vi "DatatoString.vi"(4 "Decimal Places (SI)":i32=6, 6 "Unit Modifier":enum16{"None", "RMS", "P-to-P"}(ring), 7 "SI Notation":bool, 9 "Units":string, 10 "Decimal Places (non-SI)":i32, 11 "Number":dbl format="%.6p") -> (3 "String":string)   [LabVIEW 2011]
panel:
  out "String 2":string
  # "P-to-P: Peak-to-Peak"
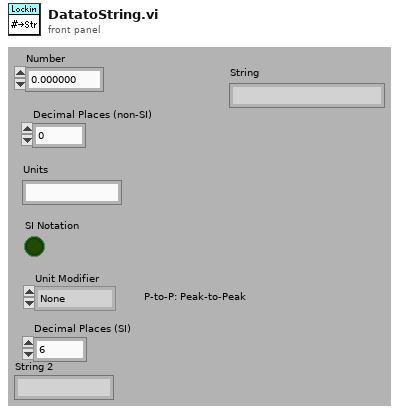
[diagram p1: front panel]
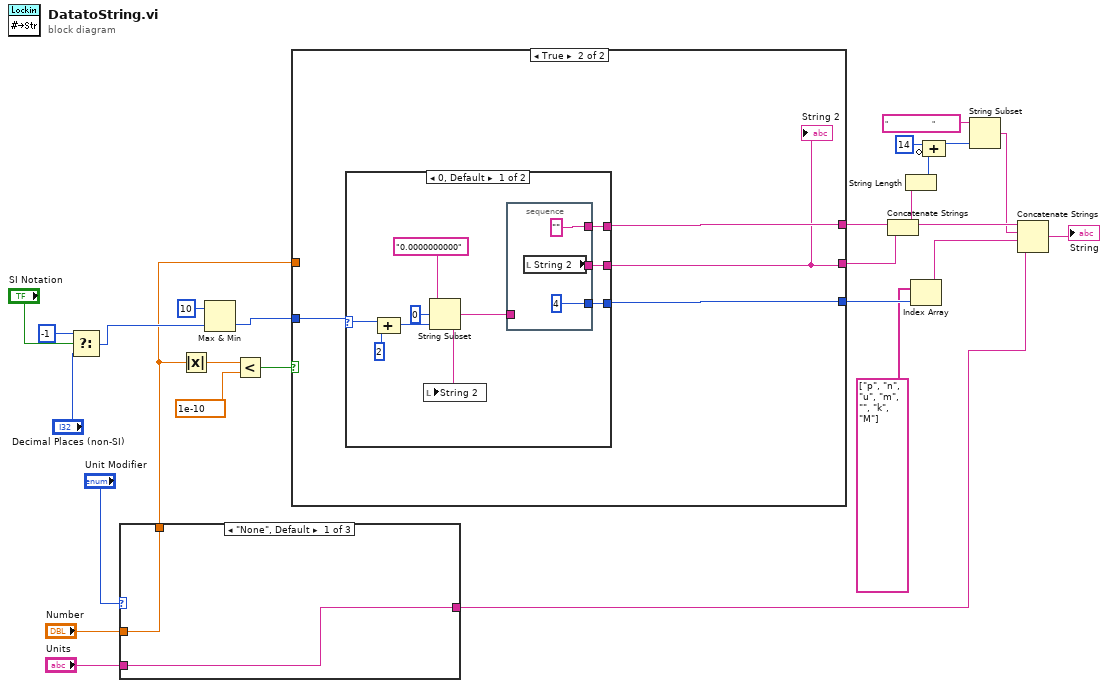
[diagram p0: block diagram]
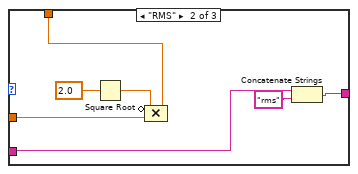
[diagram p2: hidden frame]
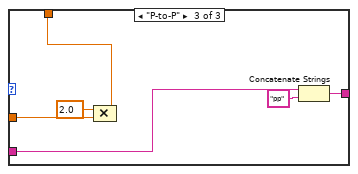
[diagram p3: hidden frame]
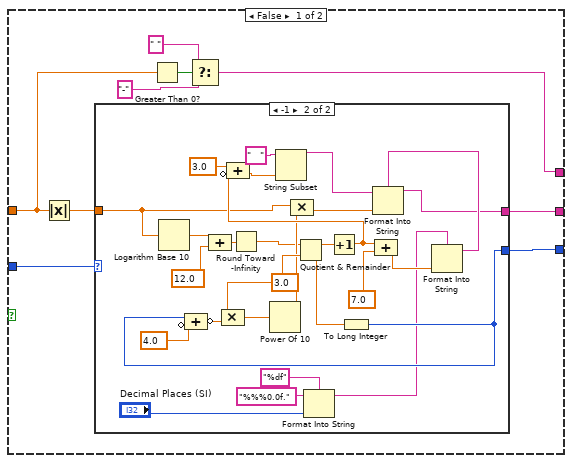
[diagram p4: hidden frame]
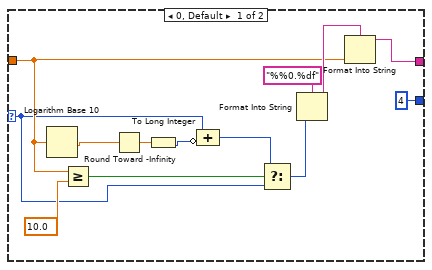
[diagram p5: hidden frame]
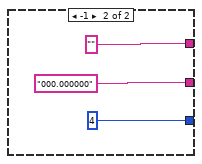
[diagram p6: hidden frame]
diagram:
  n1 = Select(t=-1, s="SI Notation", f="Decimal Places (non-SI)") -> (s? t:f=w7:i32)
  n2 = case shown="\"None\", Default" "Unit Modifier" {
    tunnel: "Number" -> [w28 w35 w41]
    tunnel: [w28 w32 w39] -> w4
    tunnel: [w27 w31 w38] -> w3
    tunnel: "Units" -> [w27 w30 w37]
    frame "None", Default {
    }
    frame "RMS" {
      n3 = Square Root(x=2.0) -> (sqrt(x)=w34:dbl)
      n4 = Compound Arithmetic op=MULTIPLY(invert w34, w35) -> (w32:dbl)
      n5 = Concatenate Strings(w30, "rms" ("string")) -> (w31:string)
    }
    frame "P-to-P" {
      n6 = Compound Arithmetic op=MULTIPLY(2.0 ("value"), w41) -> (w39:dbl)
      n7 = Concatenate Strings(w37, "pp" ("string")) -> (w38:string)
    }
  }
  n8 = Absolute Value(x=w4) -> (abs(x)=w25:dbl)
  n9 = Max & Min(x=10, y=w7) -> (min(x,y)=w12:i32)  [unwired: 1 out]
  n10 = Less?(x=w25, y=1e-10) -> (x < y?=w26:bool)
  n11 = case shown="True" w26 {
    tunnel: w12 -> [w50 w94]
    tunnel: w4 -> [w49 _]
    tunnel: [w45 w93] -> w23
    tunnel: [w43 w92] -> w16
    tunnel: [w42 w91] -> w1
    frame False {
      n12 = Absolute Value(x=w49) -> (abs(x)=w44:dbl)
      n13 = case shown="-1" w50 {
        selector: w50 -> [w55 _]
        tunnel: w44 -> [w58 w77]
        tunnel: [4 w70] -> w43
        tunnel: [w51 w64] -> w42
        frame 0, Default {
          n14 = Logarithm Base 10(1:w58) -> (0:w52:dbl)
          n15 = Greater Or Equal?(x=w58, y=10.0) -> (x >= y?=w59:bool)
          n16 = Round Toward -Infinity(1:w52) -> (0:w57:dbl)
          n17 = To Long Integer(number=w57) -> (32bit integer=w56:i32)
          n18 = Compound Arithmetic op=ADD(w55, invert w56) -> (w54:i32)
          n19 = Select(t=w54, s=w59, f=w55) -> (s? t:f=w53:i32)
          n20 = Format Into String(format string="%%0.%df", w53) -> (resulting string=w61:string)  [unwired: 2 in, 1 out]
          n21 = Format Into String(format string=w61, w58) -> (resulting string=w51:string)  [unwired: 2 in, 1 out]
        }
        frame -1 {
          w89 = 3.0 ("y")
          n22 = Logarithm Base 10(1:w77) -> (0:w72:dbl)
          n23 = Compound Arithmetic op=ADD(w72, 12.0 ("value")) -> (w90:dbl)
          n24 = Round Toward -Infinity(1:w90) -> (0:w71:dbl)
          n25 = Quotient & Remainder(x=w71, y=w89) -> (x-y*floor(x/y)=w88:dbl, floor(x/y)=w84:dbl)
          n26 = Format Into String(format string="%df", initial string="%%%0.0f." ("format string"), "Decimal Places (SI)") -> (resulting string=w65:string)  [unwired: 1 in, 1 out]
          n27 = Increment(x=w88) -> (x+1=w82:dbl)
          n28 = Compound Arithmetic op=ADD(3.0 ("value"), invert w82) -> (w80:dbl)
          n29 = String Subset(string="   ", length (rest)=w80) -> (substring=w78:string)  [unwired: 1 in]
          n30 = To Long Integer(number=w84) -> (32bit integer=w70:i32)
          n31 = Compound Arithmetic op=unknown(w70, invert 4.0 ("value")) -> (invert w74:dbl)
          n32 = Compound Arithmetic op=MULTIPLY(w89, w74) -> (w69:dbl)
          n33 = Power Of 10(x=w69) -> (10^x=w76:dbl)
          n34 = Compound Arithmetic op=MULTIPLY(w77, w76) -> (w75:dbl)
          n35 = Compound Arithmetic op=ADD(w82, 7.0 ("value")) -> (w86:dbl)
          n36 = Format Into String(format string=w65, w86) -> (resulting string=w85:string)  [unwired: 2 in, 1 out]
          n37 = Format Into String(format string=w85, initial string=w78, w75) -> (resulting string=w64:string)  [unwired: 1 in, 1 out]
        }
      }
      n38 = Greater Than 0?(x=w49) -> (x > 0?=w48:bool)
      n39 = Select(t=" ", s=w48, f="-") -> (s? t:f=w45:string)
    }
    frame True {
      n40 = case shown="0, Default" w94 {
        selector: w94 -> [w103 _]
        tunnel: [w95 "000.000000"] -> w91
        tunnel: [w97 ""] -> w93
        tunnel: [w99 4] -> w92
        frame 0, Default {
          n41 = Compound Arithmetic op=ADD(w103, 2 ("Input")) -> (w101:i32)
          n42 = String Subset(string="0.0000000000", offset (0)=0, length (rest)=w101) -> (substring=w96:string)
          n43 = local write "String 2"(w96) -> ()
          n44 = stacked-sequence {
            tunnel: [4] -> w99
            tunnel: [""] -> w97
            tunnel: [w104] -> w95
            tunnel: w96 -> [_]
            frame #0 {
              n45 = local read "String 2"() -> (w104:string)
            }
          }
        }
        frame -1 {
        }
      }
      "String 2" <- w91
    }
  }
  n46 = Concatenate Strings(w23, w1) -> (w18:string)
  n47 = String Length(string=w18) -> (length=w22:i32)
  n48 = Index Array(array=string[] ["p", "n", "u", "m", "", "k", "M"], index=w16) -> (element=w14:string)
  n49 = Compound Arithmetic op=ADD(14 ("value"), invert w22) -> (w20:i32)
  n50 = String Subset(string="                      ", length (rest)=w20) -> (substring=w17:string)  [unwired: 1 in]
  n51 = Concatenate Strings(w18, w17, w14, w3) -> (→"String":string)
